vi "Field Draw Robot.vi"(0 "Offset":T15, 1 "picture in":picture, 3 "Draw Number":bool, 5 "Robot":refnum<class "Robot.lvclass">, 9 "Scale mm/pixel":sgl, 11 "color(black)":u32(colorbox)=16775978, 13 "IA state":T1={"our_robots"=[], "enemy_robots"=[], "balls"=[], "geometry"={"line_width"=0, "field_length"=0, "field_width"=0, "boundary_width"=0, "referee_width"=0, "goal_width"=0, "goal_depth"=0, "goal_wall_width"=0, "center_circle_radius"=0, "defense_radius"=0, "defense_stretch"=0, "free_kick_from_defense_dist"=0, "penalty_spot_from_field_line_dist"=0, "penalty_line_from_spot_dist"=0}, "IA Judge"={"stage"="", "command"="", "our_goalie_id"=0.0, "enemy_goalie_id"=0.0, "command enum"=enum."Halt", "Time"=enum."Azul"}, "Received Timestamp"=timestamp(0 s since 1904-01-01), "Events"={"Touch"=FALSE, "Ball out"=FALSE, "id touch"=0.0, "Ball out of \nVision"=FALSE, "Ball inside \nGoalie area"=FALSE, "Robot not responding"=FALSE, "Robots responding status"=[1.0, 1.0, 1.0, 1.0, 1.0, 1.0], "Enemy Ball \nPossession"=FALSE, "Pass State"=FALSE, "id end of pass"=0.0, "Kick"=FALSE, "Id ini Possession"=0.0, "Ball Possesion"=FALSE, "Id Possesion"=0.0, "Direct Kick"=FALSE, "2nd Strk Ativo"=FALSE}}, 14 "color":enum16{"Azul", "Amarelo"}(ring), 15 "Draw Targets?":T12) -> (4 "picture out":picture)   [LabVIEW 2018]
uses:
  <vilib>/Utility/miscctls.llb/LVBoundsTypeDef.ctl
  DrawTargets.ctl
  sslview/Core/AI Input.ctl
  sslview/Core/AI Robot.ctl
  sslview/Intel/Functions Enum.ctl
  sslview/Intel/AttackerStates.ctl
  sslview/Path Planning/RRT/PathDests.ctl
  sslview/Path Planning/RRT/PathDest.ctl
  sslview/Core/AI Ball.ctl
  sslview/Core/Field Size.ctl
  sslview/Core/AI Judge.ctl
  sslview/Intel/Command Enum.ctl
  sslview/Util/Events/Events.ctl
  Robot_class/Robot.lvclass
  C:/Users/nicolas.oliveira/roboime/SSL_AI/Object_class/Object.lvclass
  Robot_class/Robot.lvclass/Robot.ctl
  Object_class/Object.lvclass/Object.ctl
  <vilib>/Analysis/coordinate.llb/2D Cartesian Coordinate Rotation (Scalar).vi
  Object_class/Read x.vi
  Object_class/Read y.vi
  Robot_class/Read orientation.vi
  Robot_class/Read id.vi
  Robot_class/Read kick_x.vi
  <vilib>/Analysis/NI_AALPro.lvlib
panel:
  in  "pen Chute":T13={"Width"=3, "Style"=enum."Solid"}
  in  "pen":T14={"Width"=1.0, "Style"=enum."Solid"}
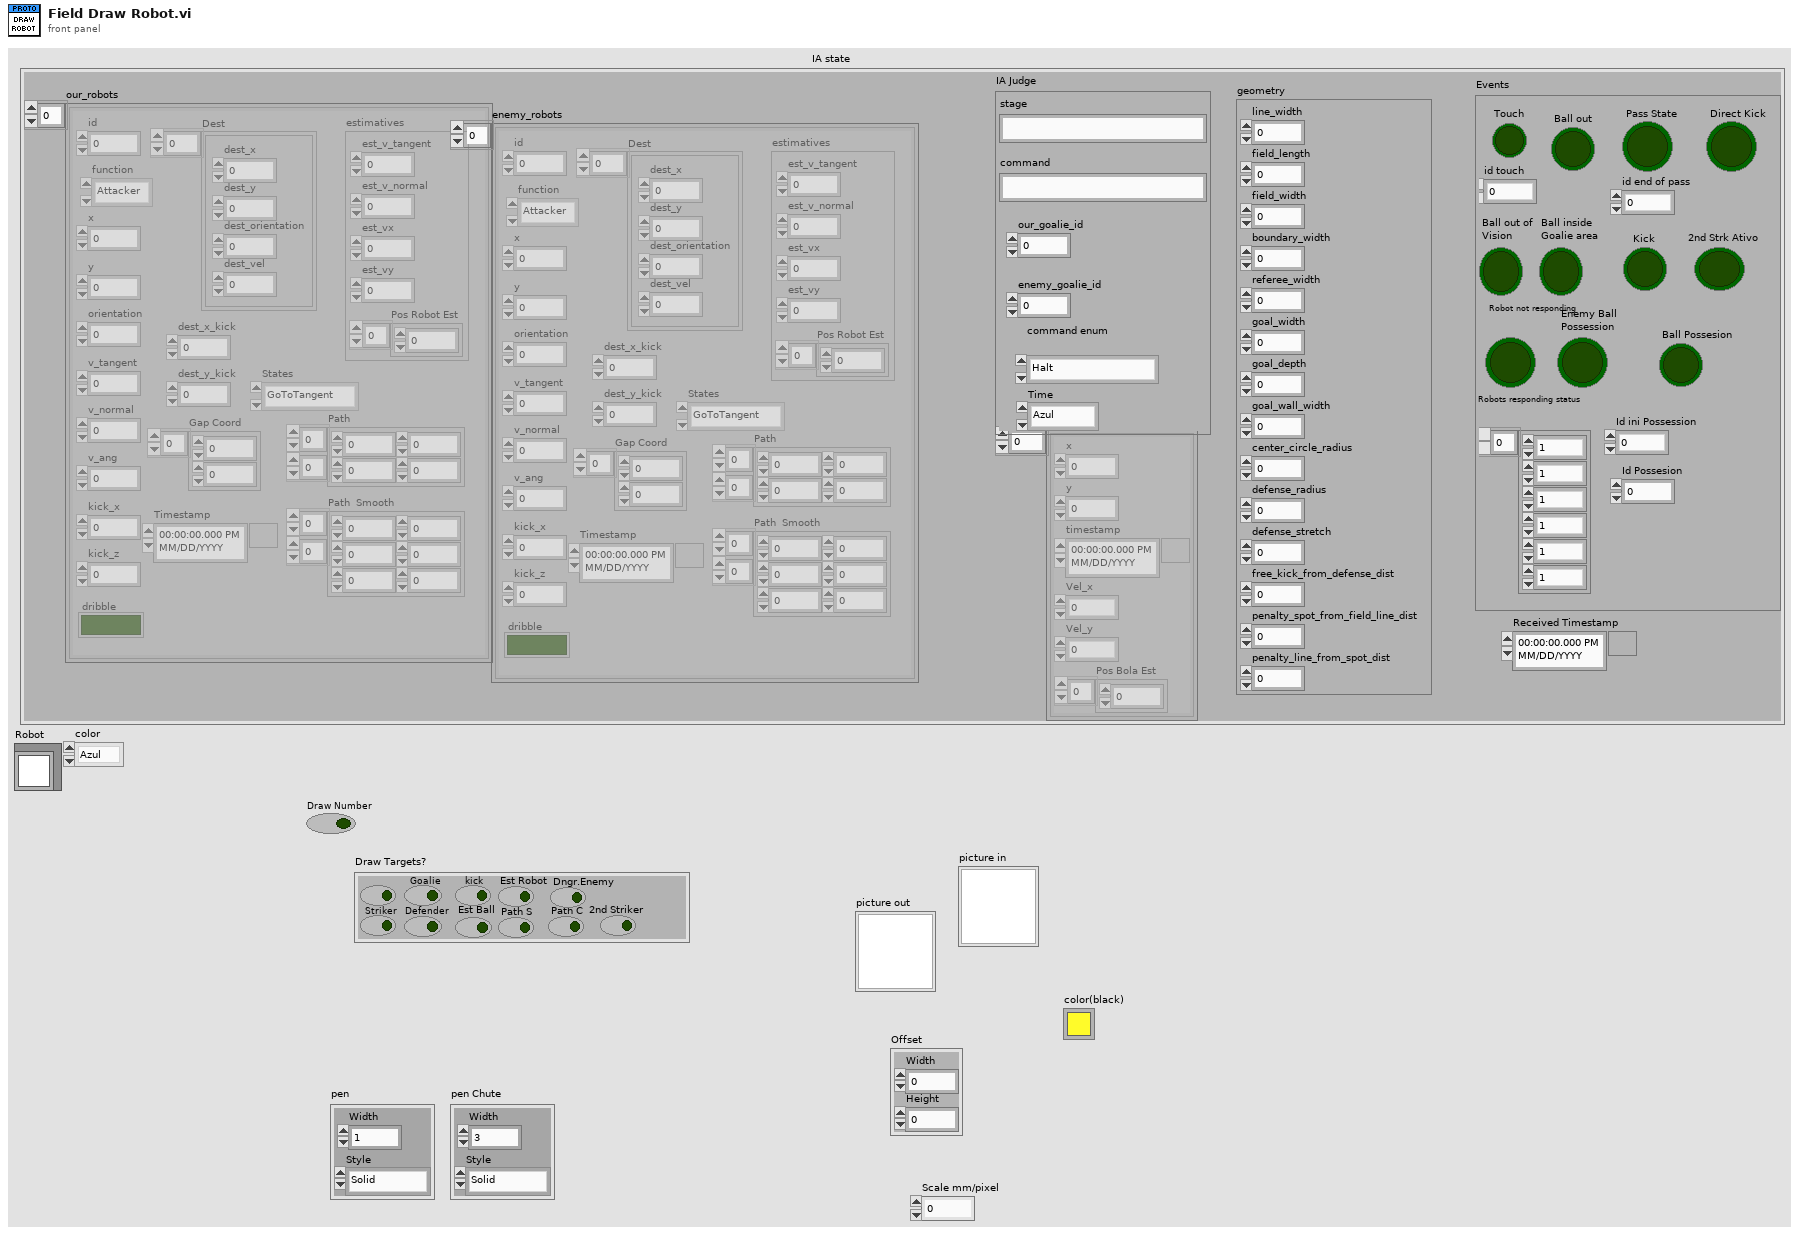
[diagram p1: front panel]
types:
  T1 = typedef "AI Input.ctl" = cluster{"our_robots":T2[], "enemy_robots":T2[], "balls":T7[], "geometry":T8, "IA Judge":T9, "Received Timestamp":timestamp, "Events":T11}
  T2 = typedef "AI Robot.ctl" = cluster{"id":u32, "function":T3, "x":dbl, "y":dbl, "orientation":dbl, "v_tangent":dbl, "v_normal":dbl, "v_ang":dbl, "kick_x":dbl, "kick_z":dbl, "dribble":bool, "Timestamp":timestamp, "estimatives":cluster{"est_v_tangent":dbl, "est_v_normal":dbl, "est_vx":dbl, "est_vy":dbl, "Pos Robot Est":dbl[]}, "dest_x_kick":dbl, "dest_y_kick":dbl, "Gap Coord":dbl[], "States":T4, "Path ":dbl[][], "Path  Smooth":dbl[][], "Dest":T5}
  T3 = typedef "Functions Enum.ctl" = enum16{"2nd Striker", "Attacker", "Goalie", "Defender", "Striker", "Goto 0", "Dummy", "Kicker", "ZigZag 0", "ZigZag 1", "ZigZag 2", "ZigZag 3", "ZigZag 4", "ZigZag 5", "ZigZag 6", "ZigZag 7", "ZigZag 8", ""}
  T4 = typedef "AttackerStates.ctl" = enum16{"Pass", "GoToTangent", "BallGetting", "GoToKick", ""}
  T5 = typedef "PathDests.ctl" = T6[]
  T6 = typedef "PathDest.ctl" = cluster{"dest_x":dbl, "dest_y":dbl, "dest_orientation":dbl, "dest_vel":dbl}
  T7 = typedef "AI Ball.ctl" = cluster{"x":dbl, "y":dbl, "timestamp":timestamp, "Vel_x":dbl, "Vel_y":dbl, "Pos Bola Est":dbl[]}
  T8 = typedef "Field Size.ctl" = cluster{"line_width":u32, "field_length":u32, "field_width":u32, "boundary_width":u32, "referee_width":u32, "goal_width":u32, "goal_depth":u32, "goal_wall_width":u32, "center_circle_radius":u32, "defense_radius":u32, "defense_stretch":u32, "free_kick_from_defense_dist":u32, "penalty_spot_from_field_line_dist":u32, "penalty_line_from_spot_dist":u32}
  T9 = typedef "AI Judge.ctl" = cluster{"stage":string, "command":string, "our_goalie_id":dbl, "enemy_goalie_id":dbl, "command enum":T10, "Time":enum16{"Azul", "Amarelo"}}
  T10 = typedef "Command Enum.ctl" = enum16{"Halt", "Stop", "Force Start", "PKA Normal Start", "Prepare Kickoff Ally", "PKE Normal Start", "Prepare Kickoff Enemy", "Prepare Penalty Ally", "PPA Normal Start", "Prepare Penalty Enemy", "PPE Normal Start", "Direct Free Enemy", "Direct Free Ally", "Indirect Free Enemy", "Indirect Free Ally", "Timeout Enemy", "Timeout Ally", "Goal Enemy", "Goal Ally", "Ball Placement Enemy", "Ball Placement Ally", "Normal Half Time", "Extra Time Break", "Extra Half Time", "None", "Post Game"}
  T11 = typedef "Events.ctl" = cluster{"Touch":bool, "Ball out":bool, "id touch":dbl, "Ball out of \nVision":bool, "Ball inside \nGoalie area":bool, "Robot not responding":bool, "Robots responding status":dbl[], "Enemy Ball \nPossession":bool, "Pass State":bool, "id end of pass":dbl, "Kick":bool, "Id ini Possession":dbl, "Ball Possesion":bool, "Id Possesion":dbl, "Direct Kick":bool, "2nd Strk Ativo":bool}
  T12 = typedef "DrawTargets.ctl" = cluster{"Attacker":bool, "Striker":bool, "Goalie":bool, "Defender":bool, "kick":bool, "Est Ball":bool, "Est Robot":bool, "Path S":bool, "Path C":bool, "Dngr.Enemy":bool, "2nd Striker":bool}
  T13 = cluster{"Width":u16, "Style":enum32{"Solid", "Dash", "Dot", "DashDot", "DashDotDot"}}
  T14 = cluster{"Width":dbl, "Style":enum32{"Solid", "Dash", "Dot", "DashDot", "DashDotDot"}}
  T15 = typedef "LVBoundsTypeDef.ctl" = cluster{"Width":u32, "Height":u32}
  T16 = cluster{"horizontal":enum16{"left", "center", "right"}, "vertical":enum16{"top", "center", "bottom"}}
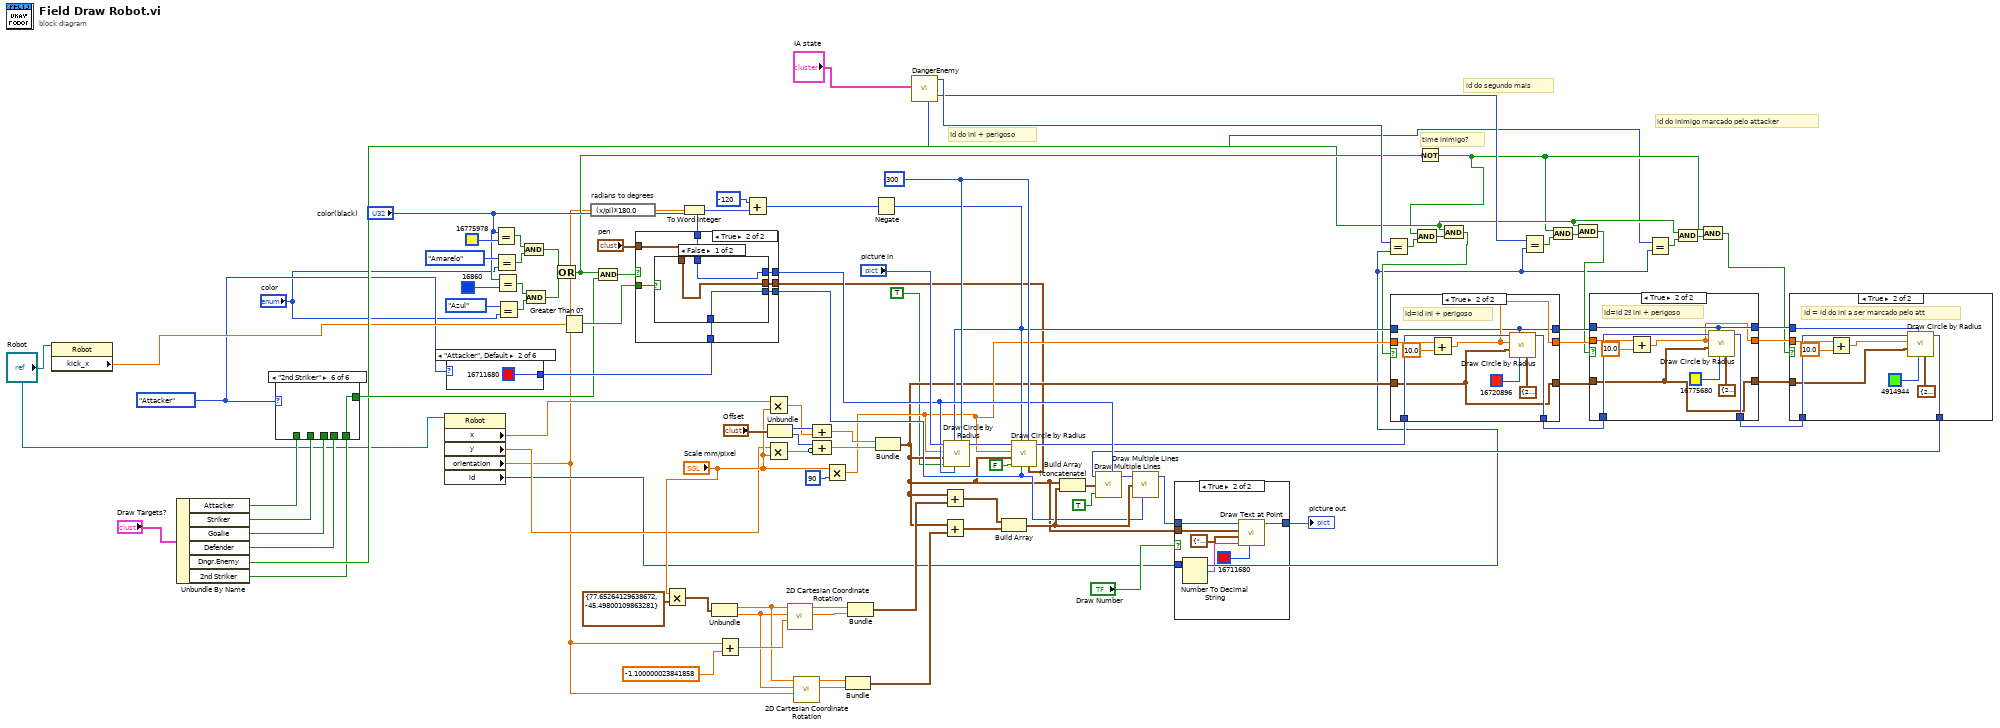
[diagram p0: block diagram]
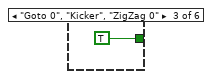
[diagram p7: hidden frame]
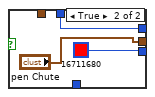
[diagram p11: hidden frame]
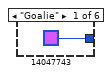
[diagram p12: hidden frame]
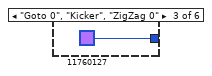
[diagram p13: hidden frame]
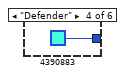
[diagram p14: hidden frame]
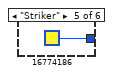
[diagram p15: hidden frame]
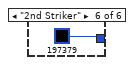
[diagram p16: hidden frame]
diagram:
  w2 = Functions_Enum."Attacker" ("function")
  w88 = i16 300 ("arc size(360)")
  # "id do inimigo marcado pelo attacker"
  # "id do segundo mais"
  # "time inimigo?"
  # "Id do ini + perigoso"
  n1 = property class="Robot"(reference="Robot") -> ("kick_x"=w3:dbl)  [unwired: 1 in, 2 out]
  n2 = Unbundle By Name("Draw Targets?") -> ("Attacker"=w47:bool, "Striker"=w46:bool, "Goalie"=w45:bool, "Defender"=w44:bool, "Dngr.Enemy"=w13:bool, "2nd Striker"=w9:bool)
  n3 = case shown="\"2nd Striker\"" w2 {
    tunnel: [w102 w103 TRUE ("Draw Target Striker?") w105 w106 w107] -> w42
    tunnel: w44 -> [_ _ _ w105 _ _]
    tunnel: w46 -> [_ _ _ _ w106 _]
    tunnel: w47 -> [w102 _ _ _ _ _]
    tunnel: w45 -> [_ w103 _ _ _ _]
    tunnel: w9 -> [_ _ _ _ _ w107]
    frame "Attacker", Default {
    }
    frame "Goalie" {
    }
    frame "Goto 0", "Kicker", "ZigZag 0" {
    }
    frame "Defender" {
    }
    frame "Striker" {
    }
    frame "2nd Striker" {
    }
  }
  n4 = property class="Robot"(reference="Robot") -> ("x"=w8:dbl, "y"=w7:dbl, "orientation"=w5:dbl, "id"=w6:i32)  [unwired: 1 in, 2 out]
  n5 = case shown="\"Attacker\", Default" w2 {
    tunnel: [u32 14047743 ("color(black)") u32 16711680 ("color(black)") u32 11760127 ("color(black)") u32 4390883 ("color(black)") u32 16774186 ("color(black)") u32 197379 ("color(black)")] -> w51
    frame "Goalie" {
    }
    frame "Attacker", Default {
    }
    frame "Goto 0", "Kicker", "ZigZag 0" {
    }
    frame "Defender" {
    }
    frame "Striker" {
    }
    frame "2nd Striker" {
    }
  }
  n6 = Equal?(x="color(black)", y=u32 16775978 ("color(black)")) -> (x = y?=w58:bool)
  n7 = Equal?(x=enum16{"Azul", "Amarelo"}."Amarelo", y="color") -> (x = y?=w59:bool)
  n8 = Equal?(x="color(black)", y=u32 16860 ("color(black)")) -> (x = y?=w55:bool)
  n9 = Equal?(x=enum16{"Azul", "Amarelo"}."Azul", y="color") -> (x = y?=w56:bool)
  n10 = And(x=w58, y=w59) -> (x .and. y?=w53:bool)
  n11 = And(x=w55, y=w56) -> (x .and. y?=w52:bool)
  n12 = Or(x=w53, y=w52) -> (x .or. y?=w24:bool)
  n13 = Greater Than 0?(x=w3) -> (x > 0?=w50:bool)
  n14 = expression code="(x/pi)*180.0" "radians to degrees"(w5) -> (w92:dbl)
  n15 = And(x=w24, y=w42) -> (x .and. y?=w43:bool)
  n16 = case shown="True" w43 {
    tunnel: [w115 w122] -> w63
    tunnel: [w115 w121] -> w62
    tunnel: "color(black)" -> [w115 w120]
    tunnel: w51 -> [_ w119]
    tunnel: [w114 w118] -> w36
    tunnel: w50 -> [_ w117]
    tunnel: "pen" -> [w114 w116]
    frame False {
    }
    frame True {
      n17 = case shown="False" w117 {
        tunnel: [w124 u32 16711680 ("color(black)")] -> w121
        tunnel: w120 -> [w125 w127]
        tunnel: [w125 w127] -> w122
        tunnel: w119 -> [w124 _]
        tunnel: [w123 "pen Chute"] -> w118
        tunnel: w116 -> [w123 _]
        frame False {
        }
        frame True {
        }
      }
    }
  }
  n18 = Multiply(x="Scale mm/pixel", y=cluster{sgl, sgl} {77.65264, -45.498} ("appended array")) -> (x*y=w70:cluster{sgl, sgl})
  n19 = To Word Integer(number=w92) -> (16bit integer=w91:i16)
  n20 = Unbundle(w70) -> (w76:sgl, w75:sgl)
  n21 = Add(x=w5, y=sgl -1.1 ("theta")) -> (x+y=w77:dbl)
  n22 = Add(x=i16 -120, y=w91) -> (x+y=w90:i16)
  n23 = Multiply(x=w8, y="Scale mm/pixel") -> (x*y=w98:dbl)
  n24 = Multiply(x=w7, y="Scale mm/pixel") -> (x*y=w95:dbl)
  n25 = Unbundle("Offset") -> ("Width"=w99:u32, "Height"=w96:u32)
  n26 = call-poly <vilib>:"2D Cartesian Coordinate Rotation.vi"("theta"=w77, "y"=w75, "x"=w76) -> ("y out"=w79:dbl, "x out"=w80:dbl)  [unwired: 6 in, 1 out]
  n27 = call-poly <vilib>:"2D Cartesian Coordinate Rotation.vi"("theta"=w5, "y"=w75, "x"=w76) -> ("y out"=w73:dbl, "x out"=w74:dbl)  [unwired: 6 in, 1 out]
  n28 = Compound Arithmetic op=ADD(w99, w98) -> (w97:dbl)
  n29 = Compound Arithmetic op=ADD(w96, invert w95) -> (w94:dbl)
  n30 = Multiply(x="Scale mm/pixel", y=i16 90 ("radius")) -> (x*y=w39:sgl)
  n31 = Bundle("x out"=w74, "y out"=w73) -> (w69:cluster{"x out":dbl, "y out":dbl})  [unwired: 1 in]
  n32 = Bundle("x out"=w80, "y out"=w79) -> (w68:cluster{"x out":dbl, "y out":dbl})  [unwired: 1 in]
  n33 = Negate(x=w90) -> (-x=w41:i16)
  n34 = Bundle(w97, w94) -> (w38:cluster{dbl, dbl})  [unwired: 1 in]
  n35 = call "DangerEnemy.vi"("IA Input"="IA state") -> ("id do segundo inimigo\nmais perigoso"=w30:i32, "id do inimigo\nmais perigoso"=w32:u32, "Id do Inimigo Mais Próximo"=w10:u32)  [unwired: 5 in, 3 out]
  n36 = Add(x=w38, y=w68) -> (x+y=w66:cluster{dbl, dbl})
  n37 = Add(x=w38, y=w69) -> (x+y=w67:cluster{dbl, dbl})
  n38 = call <vilib>:"Draw Circle by Radius.vi"("arc size(360)"=w88, "color(black)"=w63, "start angle(0)"=w41, "fill?(F)"=TRUE, "pixel center"=w38, "radius"=w39, "picture"="picture in") -> ("new picture"=w64:picture)  [unwired: 4 in]
  n39 = Build Array(w66, w67) -> (w85:cluster{dbl, dbl}[])
  n40 = call <vilib>:"Draw Circle by Radius.vi"("pen"=w36, "arc size(360)"=w88, "color(black)"=w62, "start angle(0)"=w41, "fill?(F)"=FALSE, "pixel center"=w38, "radius"=w39, "picture"=w64) -> ("new picture"=w40:picture)  [unwired: 3 in]
  n41 = Build Array (concatenate)(w38, w85) -> (w83:cluster{dbl, dbl}[])
  n42 = Equal?(x=w32, y=w6) -> (x = y?=w35:bool)
  n43 = Not(x=w24) -> (.not. x?=w12:bool)
  n44 = And(x=w12, y=w35) -> (x .and. y?=w25:bool)
  n45 = And(x=w13, y=w25) -> (x .and. y?=w23:bool)
  n46 = case shown="True" w23 {
    tunnel: w41 -> [w131 w134]
    tunnel: w40 -> [w132 w141]
    tunnel: [w132 w140] -> w29
    tunnel: w39 -> [w130 w139]
    tunnel: w38 -> [w129 w133]
    tunnel: [w131 w134] -> w28
    tunnel: [w130 w135] -> w27
    tunnel: [w129 w133] -> w26
    frame False {
    }
    frame True {
      # "Id=id ini + perigoso"
      n47 = Add(x=w139, y=sgl 10.0) -> (x+y=w135:sgl)
      n48 = call <vilib>:"Draw Circle by Radius.vi"("pen"=T13 {"Width"=2, "Style"=enum."Solid"}, "color(black)"=u32 16720896, "start angle(0)"=w134, "pixel center"=w133, "radius"=w135, "picture"=w141) -> ("new picture"=w140:picture)  [unwired: 5 in]
    }
  }
  n49 = Equal?(x=w30, y=w6) -> (x = y?=w31:bool)
  n50 = And(x=w12, y=w31) -> (x .and. y?=w22:bool)
  n51 = And(x=w13, y=w22) -> (x .and. y?=w21:bool)
  n52 = case shown="True" w21 {
    tunnel: w28 -> [w144 w148]
    tunnel: w29 -> [w145 w154]
    tunnel: [w145 w153] -> w17
    tunnel: w27 -> [w143 w152]
    tunnel: w26 -> [w142 w146]
    tunnel: [w144 w148] -> w20
    tunnel: [w143 w147] -> w19
    tunnel: [w142 w146] -> w18
    frame False {
    }
    frame True {
      # "Id=id 2º ini + perigoso"
      n53 = Add(x=w152, y=sgl 10.0) -> (x+y=w147:sgl)
      n54 = call <vilib>:"Draw Circle by Radius.vi"("pen"=T13 {"Width"=2, "Style"=enum."Solid"}, "color(black)"=u32 16775680, "start angle(0)"=w148, "pixel center"=w146, "radius"=w147, "picture"=w154) -> ("new picture"=w153:picture)  [unwired: 5 in]
    }
  }
  n55 = Equal?(x=w10, y=w6) -> (x = y?=w14:bool)
  n56 = And(x=w13, y=w14) -> (x .and. y?=w15:bool)
  n57 = And(x=w12, y=w15) -> (x .and. y?=w11:bool)
  n58 = case shown="True" w11 {
    tunnel: w20 -> [_ w164]
    tunnel: w17 -> [w155 w163]
    tunnel: [w155 w162] -> w16
    tunnel: w19 -> [_ w161]
    tunnel: w18 -> [_ w160]
    frame False {
    }
    frame True {
      # "Id = id do ini a ser marcado pelo att"
      n59 = Add(x=w161, y=sgl 10.0) -> (x+y=w159:sgl)
      n60 = call <vilib>:"Draw Circle by Radius.vi"("pen"=T13 {"Width"=2, "Style"=enum."Solid"}, "color(black)"=u32 4914944, "start angle(0)"=w164, "pixel center"=w160, "radius"=w159, "picture"=w163) -> ("new picture"=w162:picture)  [unwired: 5 in]
    }
  }
  n61 = call <vilib>:"Draw Multiple Lines.vi"("picture"=w16, "line endpoints"=w83, "fill?(F)"=TRUE, "color(black)"=w63) -> ("new picture"=w84:picture)  [unwired: 5 in]
  n62 = call <vilib>:"Draw Multiple Lines.vi"("picture"=w84, "line endpoints"=w85, "color(black)"=w62) -> ("new picture"=w86:picture)  [unwired: 6 in]
  n63 = case shown="True" "Draw Number" {
    tunnel: [w165 w172] -> w89
    tunnel: w6 -> [_ w170]
    tunnel: w86 -> [w165 w168]
    tunnel: w38 -> [_ w167]
    frame False {
    }
    frame True {
      n64 = Number To Decimal String(number=w170) -> (decimal integer string=w171:string)  [unwired: 1 in]
      n65 = call <vilib>:"Draw Text at Point.vi"("text color(black)"=u32 16711680, "text"=w171, "alignment(left, top)"=T16 {"horizontal"=enum."center", "vertical"=enum."center"}, "origin"=w167, "picture"=w168) -> ("new picture"=w172:picture)  [unwired: 5 in, 1 out]
    }
  }
  "picture out" <- w89
